vi "APU FXP Speed to DBL Speed.vi"(11 "FXP speed":fxp<+/-,23,2>) -> (3 "DBL speed":dbl)   [LabVIEW 2020, in "Engine Simulation Toolkit Engine.lvlib"]
uses:
  Engine Simulation Toolkit Engine.lvlib
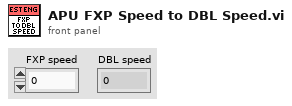
[diagram p1: front panel]
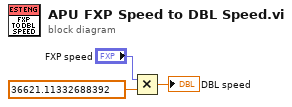
[diagram p0: block diagram]
diagram:
  n1 = Multiply(x="FXP speed", y=36621.11332688392) -> (x*y=→"DBL speed":dbl)
